vi "Database.Main.CheckIfVariantsNeedUpdate.vi"(8 "error in (no error)":errorcluster, 11 "i":i32) -> (0 "error out":errorcluster)   [LabVIEW 2016]
uses:
  Databaser.SelectVariant.Format.ctl
  Global/ApplicationGlobal.vi
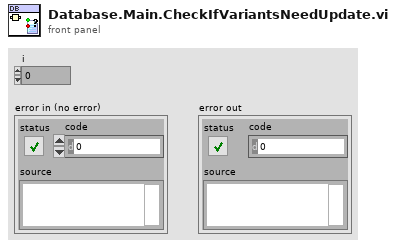
[diagram p1: front panel]
types:
  T1 = typedef "Databaser.SelectVariant.Format.ctl" = cluster{"System":string, "Variant":string}
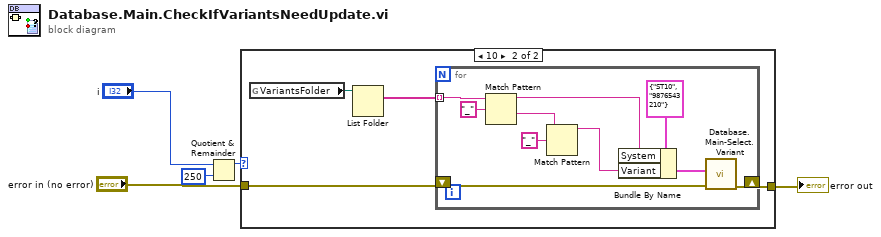
[diagram p0: block diagram]
diagram:
  n1 = Quotient & Remainder(x="i", y=250) -> (x-y*floor(x/y)=w5:i32)  [unwired: 1 out]
  n2 = case shown="10" w5 {
    tunnel: "error in (no error)" -> [w6 w10]
    tunnel: [w6 w9] -> w2
    frame 0, Default {
    }
    frame 10 {
      n3 = global read "ApplicationGlobal.vi" "VariantsFolder"() -> (w8:path)
      n4 = List Folder(path=w8) -> (filenames=w7:string[])  [unwired: 3 in, 3 out]
      n5 = for {
        shift-right: [w19] -> w9
        shift-left: w10 -> [w20]
        tunnel: w7 -> [w18] mode=indexing
        n6 = Match Pattern(string=w18, regular expression="_") -> (before substring=w13:string, after substring=w15:string)  [unwired: 1 in, 2 out]
        n7 = Match Pattern(string=w15, regular expression="_") -> (before substring=w12:string)  [unwired: 1 in, 3 out]
        n8 = Bundle By Name(cluster=T1 {"System"="ST10", "Variant"="9876543210"} ("Cluster"), "System"=w13, "Variant"=w12) -> (w11:T1)
        n9 = call "Database.Main-Select.Variant.vi"("error in"=w20, "SelectVariant Format"=w11) -> ("error out"=w19:errorcluster)  [unwired: 9 in]
      }
    }
  }
  "error out" <- w2
